vi "Enable  Disable Controls.vi"() -> ()   [LabVIEW 2019]
panel:
  in  "Array":refnum<vi>[](array[refnum])
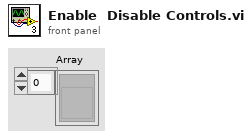
[diagram p1: front panel]
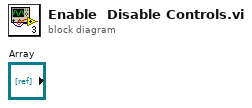
[diagram p0: block diagram]
diagram:
